vi "StartVI.vi"(11 "error in":errorcluster) -> (4 "Application Ref out":refnum<vi>, 6 "VI Reference":refnum<vi>, 15 "error out":errorcluster)   [LabVIEW 2016, in "Car Wash Test.lvlib"]
uses:
  Car Wash Test.lvlib
  APIs/Get/GetVI/GetVIByName.vi
  APIs/Stimulus/VI/RunVI.vi
  APIs/Stimulus/VI/OpenVIFrontPanel.vi
  APIs/Stimulus/VI/MakeVIFrontMost.vi
  Drona.lvlib
  APIs/Get/GetVI/GetVI.lvlib
  apis/Stimulus/VI/VI.lvlib
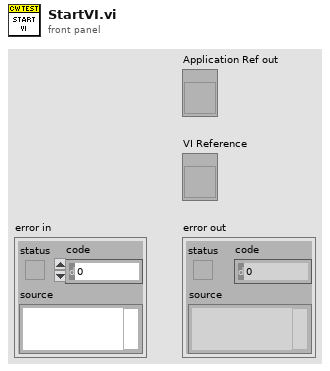
[diagram p1: front panel]
types:
  T1 = enum32{"Bad", "Idle", "Run top level", "Running"}
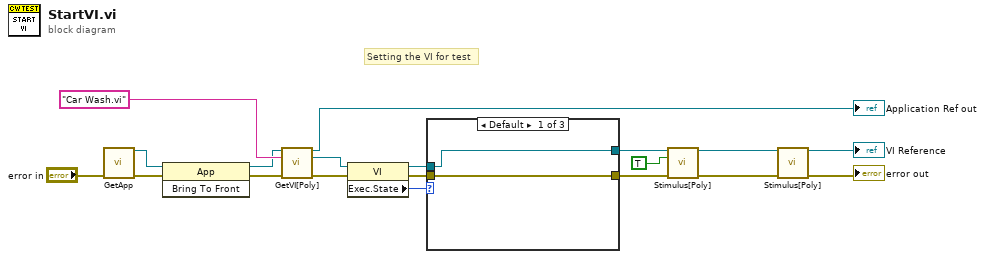
[diagram p0: block diagram]
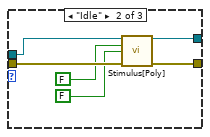
[diagram p2: hidden frame]
diagram:
  # "Setting the VI for test"
  n1 = call "GetApp.vi"("error in (no error)"="error in") -> ("Application Ref"=w4:refnum<vi>, "error out"=w2:errorcluster)  [unwired: 13 in]
  n2 = invoke class="App" method="Bring To Front"(reference=w4, error in=w2) -> (reference out=w3:refnum<vi>, error out=w1:errorcluster)  [unwired: 1 in, 1 out]
  n3 = call-poly "GetVI[Poly].vi"("Application Ref in"=w3, "VI Name"="Car Wash.vi", "error in (no error)"=w1) -> ("Application Ref out"=→"Application Ref out":refnum<vi>, "VI Reference"=w16:refnum<vi>, "error out"=w6:errorcluster)  [unwired: 10 in]
  n4 = property class="VI"(reference=w16, error in=w6) -> (reference out=w14:refnum<vi>, error out=w17:errorcluster, "Exec.State"=w15:T1)
  n5 = case shown="Default" w15 {
    tunnel: [w20 w25 w29] -> w13
    tunnel: [w21 w26 w28] -> w12
    tunnel: w17 -> [w20 w24 w29]
    tunnel: w14 -> [w21 w27 w28]
    frame Default {
    }
    frame "Idle" {
      n6 = call-poly "Stimulus[Poly].vi"("VI Reference In"=w27, "Wait Until Done (F)"=FALSE ("Wait Until Done"), "Auto Dispose Reference (F)"=FALSE ("Auto Dispose Reference"), "error in"=w24) -> ("VI Reference Out"=w26:refnum<vi>, "error out"=w25:errorcluster)  [unwired: 10 in]
    }
    frame "Run top level", "Running" {
    }
  }
  n7 = call-poly "Stimulus[Poly].vi"("VI Reference In"=w12, "Wait Until Done (F)"=TRUE, "error in"=w13) -> ("VI Reference Out"=w9:refnum<vi>, "error out"=w10:errorcluster)  [unwired: 11 in]
  n8 = call-poly "Stimulus[Poly].vi"("VI Reference In"=w9, "error in"=w10) -> ("VI Reference Out"=→"VI Reference":refnum<vi>, "error out"=→"error out":errorcluster)  [unwired: 12 in]
